vi "p30_3_rpy.vi"() -> ()   [LabVIEW 2013]
panel:
  out "gamma (RPY)":cluster{"roll":dbl, "pitch":dbl, "yaw":dbl}
  out "transformation matrix":picture
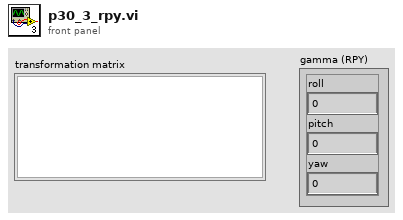
[diagram p1: front panel]
types:
  T1 = typedef "NI_Matrix.lvlib/RealMatrix.ctl" = dbl[][]
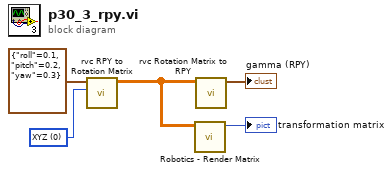
[diagram p0: block diagram]
diagram:
  w3 = u16 0 items=["XYZ", "ZYX"] ("Convension")
  n1 = call "rvc RPY to Rotation Matrix.vi"("Convension"=w3, "angles"=cluster{"roll":dbl, "pitch":dbl, "yaw":dbl} {"roll"=0.1, "pitch"=0.2, "yaw"=0.3}) -> ("rotation matrix"=w1:T1)  [unwired: 9 in]
  n2 = call "Robotics - Render Matrix.vi"("A"=w1) -> ("picture out"=→"transformation matrix":picture)  [unwired: 10 in]
  n3 = call "rvc Rotation Matrix to RPY.vi"("rotation matrix"=w1) -> ("angles"=→"gamma (RPY)":cluster{"roll":dbl, "pitch":dbl, "yaw":dbl})  [unwired: 10 in]
